vi "TxtFile Load.vi"(8 "error in (no error)":errorcluster, 11 "Path":path) -> (0 "error out":errorcluster, 3 "text":string)   [LabVIEW 2017]
doc: "Reads a text file and returns its contents. A file encoded as UTF-8 is converted to text, so non-ASCII characters are read correctly."
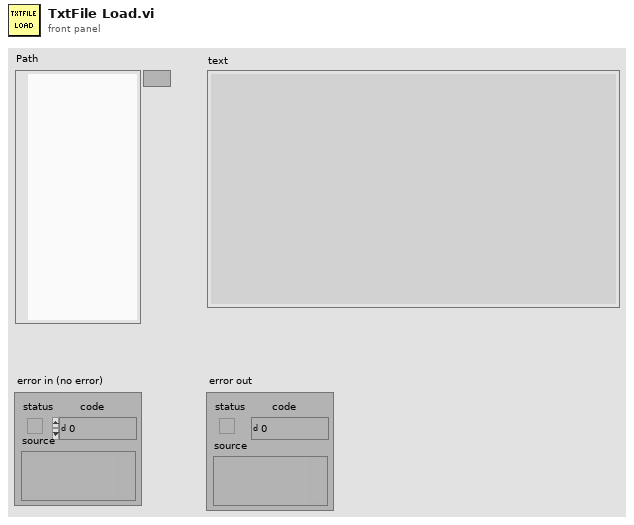
[diagram p1: front panel]
types:
  T1 = enum16{"open", "replace", "create", "open or create", "replace or create", "replace or create with confirmation"}
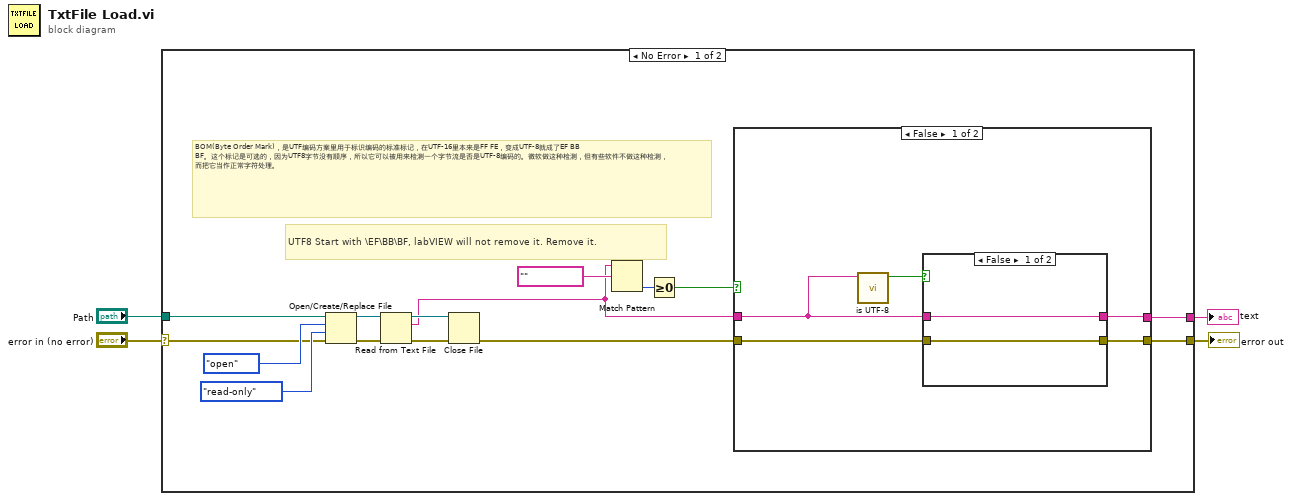
[diagram p0: block diagram]
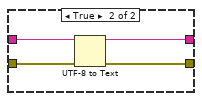
[diagram p2: hidden frame]
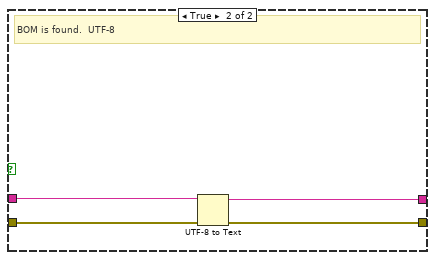
[diagram p3: hidden frame]
diagram:
  n1 = case shown="No Error" "error in (no error)" {
    selector: "error in (no error)" -> [w7 w35]
    tunnel: [w8 w35] -> w3
    tunnel: "Path" -> [w6 _]
    tunnel: [w13 _] -> w1
    frame No Error {
      # "BOM(Byte Order Mark)，是UTF编码方案里用于标识编码的标准标记，在UTF-16里本来是FF FE，变成UTF-8就成了EF BB BF。这个标记是可选的，因为UTF8字节没有顺序，所以它可以被用来检测一个字节流是否是UTF-8编码的。微软做这种检测，但有些软件不做这种检测， 而把它当作正常字符处理。"
      # "UTF8 Start with \\EF\\BB\\BF, labVIEW will not remove it. Remove it."
      n2 = Open/Create/Replace File(file path (use dialog)=w6, error in=w7, operation (0:open)=T1."open", access (0:read/write)=enum16{"read/write", "read-only", "write-only"}."read-only") -> (refnum out=w17:refnum<file>, error out=w14:errorcluster)  [unwired: 2 in, 1 out]
      n3 = Read from Text File(file (use dialog)=w17, error in=w14) -> (refnum out=w16:refnum<file>, text=w5:string, error out=w15:errorcluster)  [unwired: 2 in, 1 out]
      n4 = Close File(refnum=w16, error in=w15) -> (error out=w9:errorcluster)  [unwired: 1 out]
      n5 = Match Pattern(string=w5, regular expression="﻿") -> (offset past match=w12:i32)  [unwired: 1 in, 3 out]
      n6 = Greater Or Equal To 0?(x=w12) -> (x >= 0?=w11:bool)
      n7 = case shown="False" w11 {
        tunnel: [w23 w33] -> w13
        tunnel: w5 -> [w22 w34]
        tunnel: w9 -> [w20 w32]
        tunnel: [w21 w31] -> w8
        frame False {
          n8 = call "is UTF-8.vi"("String"=w22) -> ("UTF8"=w24:bool)  [unwired: 10 in]
          n9 = case shown="False" w24 {
            tunnel: w22 -> [w25 w30]
            tunnel: [w25 w29] -> w23
            tunnel: w20 -> [w26 w28]
            tunnel: [w26 w27] -> w21
            frame False {
            }
            frame True {
              n10 = UTF-8 to Text(8:w28, 11:w30) -> (0:w27:errorcluster, 3:w29:string)  [unwired: 1 in]
            }
          }
        }
        frame True {
          # "BOM is found.  UTF-8"
          n11 = UTF-8 to Text(8:w32, 11:w34) -> (0:w31:errorcluster, 3:w33:string)  [unwired: 1 in]
        }
      }
    }
    frame Error {
    }
  }
  "error out" <- w3
  "text" <- w1
